vi "SetI.vi"(8 "error in (no error)":errorcluster, 10 "i 3":i32, 11 "reference in":refnum<class "GOOP4_Sub.lvclass">) -> (0 "error out":errorcluster, 3 "reference in":refnum<class "GOOP4_Sub.lvclass">)   [LabVIEW 2019, in "GOOP4_Sub.lvclass"]
uses:
  GOOP4_Sub.lvclass
  GOOP4_Base_class/GOOP4_Base.lvclass
  C:/Users/Tiba/Desktop/1GOOP4_CreateObjects_Open_GDS/GOOP4_Base_class/GOOP4_Base.lvclass
panel:
  in  "i 2":i32
  in  "i":i32
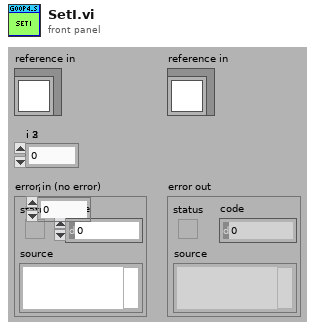
[diagram p1: front panel]
types:
  T1 = typedef "GOOP4_Base.lvclass/ObjectAttributes.ctl" = cluster{"i":i32}
  T2 = typedef "GOOP4_Sub.lvclass/ObjectAttributes.ctl" = cluster{"Str":string, "Boolean":bool}
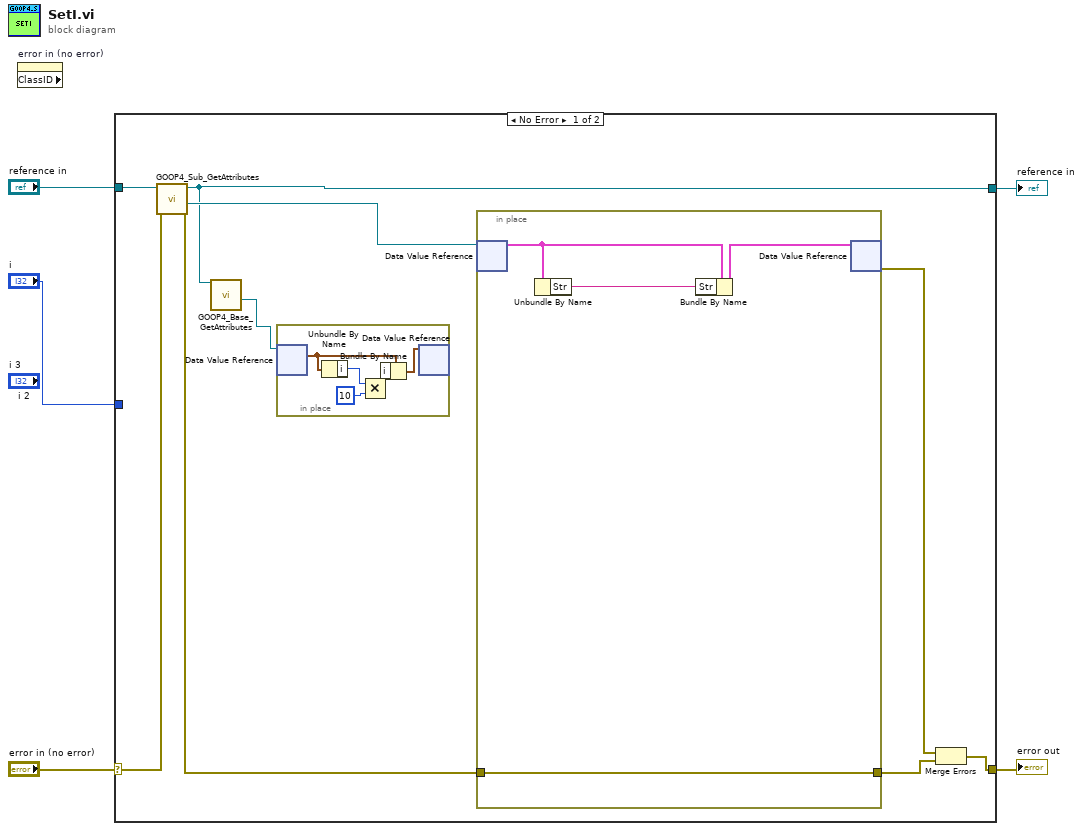
[diagram p0: block diagram]
diagram:
  n1 = property on="error in (no error)" class="Clust (strict)" props=["ClassID"]() -> ()  [unwired: 2 in, 3 out]
  n2 = case shown="No Error" "error in (no error)" {
    selector: "error in (no error)" -> [w13 w25]
    tunnel: [w11 w25] -> w4
    tunnel: [w7 w24] -> w2
    tunnel: "reference in" -> [w14 w24]
    tunnel: "i" -> [_ _]
    frame No Error {
      n3 = call "GOOP4_Sub_GetAttributes.vi"("error in (no error)"=w13, "reference in"=w14) -> ("error out"=w9:errorcluster, "DataRef"=w10:refnum<data-value>, "reference out"=w7:refnum<class "GOOP4_Sub.lvclass">)  [unwired: 6 in, 1 out]
      n4 = call "GOOP4_Base_GetAttributes.vi"("reference in"=w7) -> ("DataRef"=w6:refnum<data-value>)  [unwired: 7 in, 3 out]
      n5 = in-place {
        n6 = in-place-dvr #1(w6) -> (w15:T1)  [unwired: 1 out]
        n7 = Unbundle By Name(w15) -> ("i"=w16:i32)
        n8 = Multiply(x=w16, y=10) -> (x*y=w18:i32)
        n9 = Bundle By Name(cluster=w15, "i"=w18) -> (w17:T1)
        n10 = in-place-dvr #1(w17) -> ()  [unwired: 2 out]
      }
      n11 = in-place {
        in-place-border: w9 -> [w22]
        in-place-border: [w22] -> w8
        n12 = in-place-dvr #2(w10) -> (w21:T2)  [unwired: 1 out]
        n13 = Unbundle By Name(w21) -> ("Str"=w20:string)
        n14 = Bundle By Name(cluster=w21, "Str"=w20) -> (w23:T2)
        n15 = in-place-dvr #2(w23) -> (w12:errorcluster)  [unwired: 1 out]
      }
      n16 = Merge Errors(w12, w8) -> (w11:errorcluster)
    }
    frame Error {
    }
  }
  "error out" <- w4
  "reference in" <- w2
